vi "Test SplashWindow1.vi"() -> ()   [LabVIEW 2020]
uses:
  fedf0d60-aefe-4d5b-acf5-983cba3c9748.vi
  fedf0d60-aefe-4d5b-acf5-983cba3c9748.vi/1b47866c-8e2d-43a7-815f-8cf18635e5a1.vi
  <userlib>/_NEVSTOP/TagDB/_Support/Change Detector/TagDB dbChanged.vi
  <userlib>/_NEVSTOP/TagDB/_Support/Error/_Clear Errors.vi
  fedf0d60-aefe-4d5b-acf5-983cba3c9748.vi/1b47866c-8e2d-43a7-815f-8cf18635e5a1.vi/29b2ea6d-6d7f-4e4a-ad31-a5cb760462c7.vi
  <userlib>/_NEVSTOP/TagDB/API/TagDB-Status.vi
  <userlib>/_NEVSTOP/TagDB/_Support/Change Detector/TagDB ChangeFlag.vi
  <userlib>/_NEVSTOP/TagDB/_Support/DataAccess/_NameCacher.vi
  <userlib>/_NEVSTOP/TagDB/_Support/Error/_[error50002]Invalid DataType.vi
  <userlib>/_NEVSTOP/TagDB/_Support/Error/_[error50000]Invalid DB REF.vi
  <userlib>/_NEVSTOP/TagDB/_Support/DataAccess/TagDB Ref to DVR.vi
  <userlib>/_NEVSTOP/TagDB/_Support/URL/TRIM-BOTH-SPACE.vi
  <userlib>/_NEVSTOP/TagDB/_Support/Error/_Build Error Cluster.vi
  CSM-SplashWindow.lvlib
  <userlib>/_NEVSTOP/Communicable State Machine(CSM)/Communicable State Machine.lvlib
  <userlib>/_NEVSTOP/TagDB/Add-ons/RefManager/TagDB RefManager.lvlib
  <userlib>/_NEVSTOP/TagDB/TagDB.lvlib
panel:
  in  "Stop":bool
  # "Splash Test Launcher"
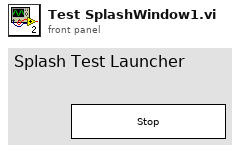
[diagram p1: front panel]
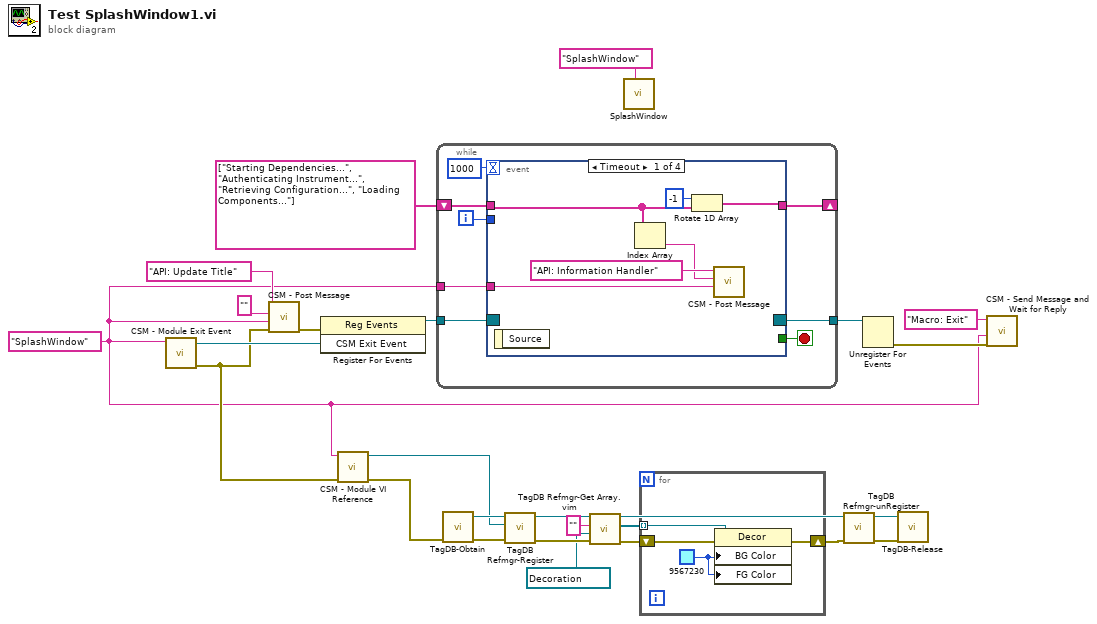
[diagram p0: block diagram]
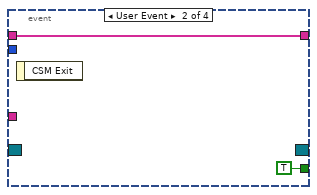
[diagram p2: hidden frame]
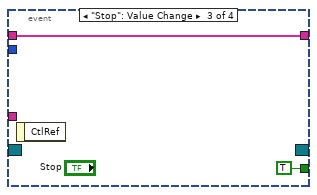
[diagram p3: hidden frame]
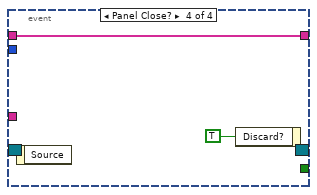
[diagram p4: hidden frame]
diagram:
  w1 = "SplashWindow" ("Name (\"\" to Use UUID)")
  n1 = call <userlib>:"CSM - Module Exit Event.vi"("Name (\"\" to Use UUID) In"=w1) -> ("error out"=w3:errorcluster, "CSM Exit Event"=w22:refnum<user-event>)  [unwired: 8 in, 1 out]
  n2 = call <userlib>:"CSM - Post Message.vi"("Error In (No Error)"=w3, "Target Module"=w1, "Arguments (\"\")"="" ("State"), "State"="API: Update Title") -> ("error out"=w18:errorcluster)  [unwired: 7 in]
  n3 = register-events(error in=w18, w22) -> (reference out=w24:refnum<event-registration>)  [unwired: 1 in, 1 out]
  n4 = call <userlib>:"CSM - Module VI Reference.vi"("error in (no error)"=w3, "CSM Name"=w1) -> ("error out"=w2:errorcluster, "CSM Module VIRef"=w15:refnum<vi>)  [unwired: 8 in]
  n5 = while {
    tunnel: w24 -> [w33]
    tunnel: [w32] -> w25
    shift-right: [w28] -> _
    shift-left: string[] ["Starting Dependencies...", "Authenticating Instrument...", "Retrieving Configuration...", "Loading Components..."] -> [w29]
    tunnel: w1 -> [w27]
    i -> [w30]
    stop <- w34 stop-if-true
    n6 = event shown="[0] Timeout" {
      selector: w33 -> [_ _ _ _]
      dyn-events: [_ _ _ _] -> w32
      timeout: 1000 -> [_ _ _ _]
      tunnel: [_ TRUE TRUE _] -> w34
      tunnel: w30 -> [_ _ _ _]
      tunnel: w29 -> [w40 w42 w44 w45]
      tunnel: [w39 w42 w44 w45] -> w28
      tunnel: w27 -> [w37 _ _ _]
      event Timeout {
        n7 = event-data() -> ()  [unwired: 1 in, 1 out]
        n8 = Index Array(array=w40) -> (element=w35:string)  [unwired: 1 in]
        n9 = Rotate 1D Array(1:w40, 2:-1 ("n")) -> (0:w39:string[])
        n10 = call <userlib>:"CSM - Post Message.vi"("Target Module"=w37, "Arguments (\"\")"=w35, "State"="API: Information Handler") -> ()  [unwired: 8 in, 1 out]
      }
      event User Event {
        n11 = event-data() -> ()  [unwired: 1 in, 1 out]
      }
      event "Stop": Value Change {
        n12 = event-data() -> ()  [unwired: 1 in, 1 out]
      }
      event Panel Close? {
        n13 = event-data() -> ()  [unwired: 1 in, 1 out]
        n14 = event-data("Discard?"=TRUE ("OK")) -> ()  [unwired: 1 in, 1 out]
      }
    }
  }
  n15 = call <userlib>:"TagDB-Obtain.vi"("error in (no error)"=w2) -> ("error out"=w14:errorcluster, "TagDB"=w16:refnum<k1>)  [unwired: 4 in, 1 out]
  n16 = call <userlib>:"TagDB Refmgr-Register.vi"("error in (no error)"=w14, "VI Refnum"=w15, "TagDB in"=w16) -> ("error out"=w12:errorcluster, "TagDB out"=w13:refnum<k1>)  [unwired: 6 in, 1 out]
  n17 = call "TagDB Refmgr-Get Array.vim"("error in (no error)"=w12, "Type"=refnum<vi> refnum, "RegExp"="", "DB Ref"=w13) -> ("error out"=w7:errorcluster, "References"=w5:refnum<vi>[], "DB Ref(dup)"=w6:refnum<k1>)  [unwired: 4 in, 1 out]
  n18 = call "SplashWindow.vi"("Name (\"\" to Use UUID)"="SplashWindow" ("Name (\"\" to Use UUID)")) -> ()  [unwired: 11 in]
  n19 = for {
    shift-right: [w49] -> w8
    shift-left: w7 -> [w50]
    tunnel: w5 -> [w48] mode=indexing
    w47 = u32 9567230 ("Colors:BG Color")
    n20 = property class="Decor"(reference=w48, error in=w50, "BG Color"=w47, "FG Color"=w47) -> (error out=w49:errorcluster)  [unwired: 1 out]
  }
  n21 = call <userlib>:"TagDB Refmgr-unRegister.vi"("error in (no error)"=w8, "TagDB in"=w6) -> ("error out"=w10:errorcluster, "TagDB out"=w9:refnum<k1>)  [unwired: 8 in]
  n22 = Unregister For Events(event registration refnum=w25) -> (error out=w21:errorcluster)  [unwired: 1 in]
  n23 = call <userlib>:"TagDB-Release.vi"("error in (no error)"=w10, "TagDB"=w9) -> ()  [unwired: 9 in, 1 out]
  n24 = call <userlib>:"CSM - Send Message and Wait for Reply.vi"("Error In (No Error)"=w21, "Target Module"=w1, "State"="Macro: Exit") -> ()  [unwired: 6 in, 3 out]
